vi "LibXML_CopyString.vi"(8 "error in":errorcluster, 9 "free pointer?":bool, 10 "string pointer":u32, 11 "length":u32) -> (0 "error out":errorcluster, 3 "lvstring":string)   [LabVIEW 2019, in "Tools.lvlib" / "LibXML.lvlib"]
doc: "Gets a string from a string pointer (U32) input."
uses:
  LibXML.lvlib
  <vilib>/Utility/error.llb/Trim Whitespace.vi
  Tools.lvlib
  dll/lXMLwrap.dll
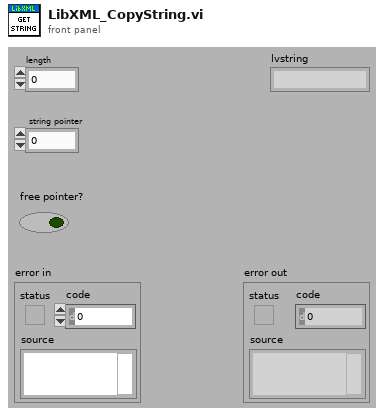
[diagram p1: front panel]
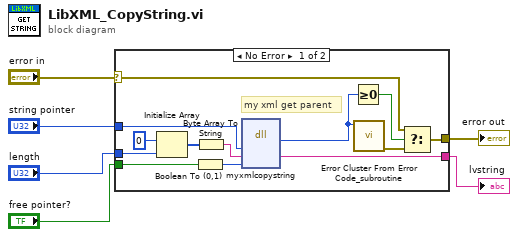
[diagram p0: block diagram]
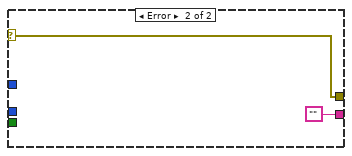
[diagram p2: hidden frame]
diagram:
  n1 = case shown="No Error" "error in" {
    selector: "error in" -> [w7 w21]
    tunnel: [w18 w21] -> w5
    tunnel: "free pointer?" -> [w11 _]
    tunnel: "length" -> [w10 _]
    tunnel: "string pointer" -> [w9 _]
    tunnel: [w8 ""] -> w1
    frame No Error {
      # "my xml get parent"
      n2 = Initialize Array(u8 0 ("element"), w10) -> (w14:u8[])
      n3 = Boolean To (0,1)(Boolean=w11) -> (0, 1=w12:i16)
      n4 = Byte Array To String(unsigned byte array=w14) -> (string=w13:string)
      n5 = dll-call lib="C:/Projects/_Prywatne/MyCIT/Framework/Tools/XML/LibXML/dll/lXMLwrap.dll" fn="myxmlcopystring"("stringptr"=w9, "lvstring"=w13, "freepointerflag"=w12) -> ("return type"=w16:u32, "lvstring"=w8:string)  [unwired: 5 in, 2 out]
      n6 = Greater Or Equal To 0?(x=w16) -> (x >= 0?=w17:bool)
      n7 = call "Error Cluster From Error Code_subroutine.vi"("error code (0)"=w16) -> ("error out"=w19:errorcluster)  [unwired: 8 in]
      n8 = Select(t=w7, s=w17, f=w19) -> (s? t:f=w18:errorcluster)
    }
    frame Error {
    }
  }
  "error out" <- w5
  "lvstring" <- w1
